vi "转换关键参数(子VI).vi"(9 "参数":u16, 10 "总磷关键参数":T2, 11 "关键参数输入":T1) -> (3 "关键参数输出":T1)   [LabVIEW 2016, in "斯坦道总磷总氮.lvlib"]
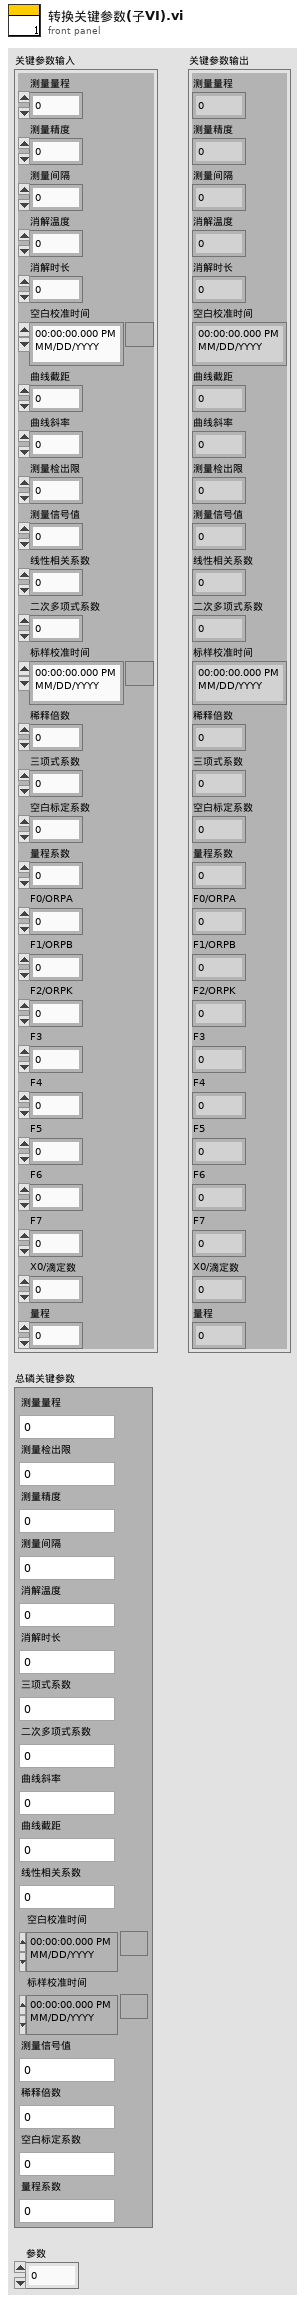
[diagram p1: front panel]
types:
  T1 = cluster{"测量量程":dbl, "测量精度":dbl, "测量间隔":dbl, "消解温度":dbl, "消解时长":dbl, "空白校准时间":timestamp, "曲线截距":dbl, "曲线斜率":dbl, "测量检出限":dbl, "测量信号值":dbl, "线性相关系数":dbl, "二次多项式系数":dbl, "标样校准时间":timestamp, "稀释倍数":dbl, "三项式系数":dbl, "空白标定系数":dbl, "量程系数":dbl, "F0/ORPA":dbl, "F1/ORPB":dbl, "F2/ORPK":dbl, "F3":dbl, "F4":dbl, "F5":dbl, "F6":dbl, "F7":dbl, "X0/滴定数":dbl, "量程":dbl}
  T2 = typedef "斯坦道总磷总氮.lvlib/关键参数.ctl" = cluster{"测量量程":sgl, "测量检出限":sgl, "测量精度":sgl, "测量间隔":sgl, "消解温度":sgl, "消解时长":sgl, "三项式系数":sgl, "二次多项式系数":sgl, "曲线斜率":sgl, "曲线截距":sgl, "线性相关系数":sgl, "空白校准时间":timestamp, "标样校准时间":timestamp, "测量信号值":sgl, "稀释倍数":sgl, "空白标定系数":sgl, "量程系数":sgl}
  T3 = cluster{"因子编码":u32, "单位":u16, "标样参考值":sgl, "水样数据时间":timestamp, "水样实测值":sgl, "水样数据标识":string, "标样数据时间":timestamp, "标样实测值":sgl, "标样数据标识":string, "空白数据时间":timestamp, "空白实测值":sgl, "空白数据标识":string, "零点核查数据时间":timestamp, "零点核查实测值":sgl, "零点核查数据标识":string, "跨度核查数据时间":timestamp, "跨度核查实测值":sgl, "跨度核查数据标识":string, "加标回收数据时间":timestamp, "加标回收实测值":sgl, "加标回收数据标识":string, "平行样数据时间":timestamp, "平行样实测值":sgl, "平行样数据标识":string, "F0":sgl, "F1":sgl, "F2":sgl, "F3":sgl, "F4":sgl, "F5":sgl, "F6":sgl, "F7":sgl, "温度":sgl, "湿度":sgl, "X值":sgl, "fidrange":u16, "X1值":sgl}[]
  T4 = cluster{"系统时间":timestamp, "工作状态":u16, "测量模式":enum16{"待机", "连续模式", "周期模式", "定点模式", "受控模式", "手动模式"}, "告警代码":u16, "故障代码":u16, "日志代码":u16, "软件版本":u16, "F0":sgl, "F1":sgl, "F2":sgl, "F3":sgl, "T":sgl, "H":sgl, "id":u16, "flowid":u16, "量程":u16, "总磷控温温度1":sgl, "营养盐控温温度2":sgl, "ADC":sgl, "结果值":sgl, "运行时间":u16, "步骤详情":string, "步骤流程":string}
  T5 = cluster{"因子编码":u32, "单位":u16, "标样参考值":sgl, "水样数据时间":timestamp, "水样实测值":sgl, "水样数据标识":string, "标样数据时间":timestamp, "标样实测值":sgl, "标样数据标识":string, "空白数据时间":timestamp, "空白实测值":sgl, "空白数据标识":string, "零点核查数据时间":timestamp, "零点核查实测值":sgl, "零点核查数据标识":string, "跨度核查数据时间":timestamp, "跨度核查实测值":sgl, "跨度核查数据标识":string, "加标回收数据时间":timestamp, "加标回收实测值":sgl, "加标回收数据标识":string, "平行样数据时间":timestamp, "平行样实测值":sgl, "平行样数据标识":string, "F0":sgl, "F1":sgl, "F2":sgl, "F3":sgl, "F4":sgl, "F5":sgl, "F6":sgl, "F7":sgl, "温度":sgl, "湿度":sgl, "X值":sgl, "fidrange":u16, "X1值":sgl}
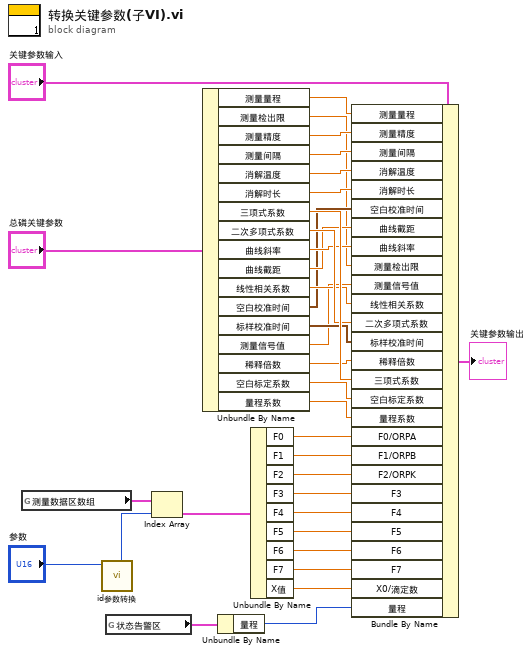
[diagram p0: block diagram]
diagram:
  n1 = global read "VAR总磷总氮全局变量.vi" "测量数据区数组"() -> (w20:T3)
  n2 = call "id参数转换.vi"("id"="参数") -> ("数组资源索引"=w21:i32)  [unwired: 9 in, 1 out]
  n3 = global read "VAR总磷总氮全局变量.vi" "状态告警区"() -> (w32:T4)
  n4 = Index Array(array=w20, index=w21) -> (element=w22:T5)
  n5 = Unbundle By Name("总磷关键参数") -> ("测量量程"=w3:sgl, "测量检出限"=w4:sgl, "测量精度"=w5:sgl, "测量间隔"=w6:sgl, "消解温度"=w7:sgl, "消解时长"=w8:sgl, "三项式系数"=w17:sgl, "二次多项式系数"=w14:sgl, "曲线斜率"=w11:sgl, "曲线截距"=w10:sgl, "线性相关系数"=w13:sgl, "空白校准时间"=w9:timestamp, "标样校准时间"=w15:timestamp, "测量信号值"=w12:sgl, "稀释倍数"=w16:sgl, "空白标定系数"=w18:sgl, "量程系数"=w19:sgl)
  n6 = Unbundle By Name(w32) -> ("量程"=w33:u16)
  n7 = Unbundle By Name(w22) -> ("F0"=w23:sgl, "F1"=w24:sgl, "F2"=w25:sgl, "F3"=w26:sgl, "F4"=w27:sgl, "F5"=w28:sgl, "F6"=w29:sgl, "F7"=w30:sgl, "X值"=w31:sgl)
  n8 = Bundle By Name(cluster="关键参数输入", "测量量程"=w3, "测量精度"=w5, "测量间隔"=w6, "消解温度"=w7, "消解时长"=w8, "空白校准时间"=w9, "曲线截距"=w10, "曲线斜率"=w11, "测量检出限"=w4, "测量信号值"=w12, "线性相关系数"=w13, "二次多项式系数"=w14, "标样校准时间"=w15, "稀释倍数"=w16, "三项式系数"=w17, "空白标定系数"=w18, "量程系数"=w19, "F0/ORPA"=w23, "F1/ORPB"=w24, "F2/ORPK"=w25, "F3"=w26, "F4"=w27, "F5"=w28, "F6"=w29, "F7"=w30, "X0/滴定数"=w31, "量程"=w33) -> (→"关键参数输出":T1)
